vi "InsertBus.vi"(8 "ErrorArray In":errorcluster[](array[cluster]), 11 "BusClass In":refnum<class "Bus.lvclass">) -> (0 "ErrorArray Out":errorcluster[](array[cluster]), 3 "BusClass Out":refnum<class "Bus.lvclass">)   [LabVIEW 2014, in "Bus_class.lvlib" / "Bus.lvclass"]
uses:
  Bus.lvclass
  Bus.lvclass/Bus.ctl
  Framework.lvlib
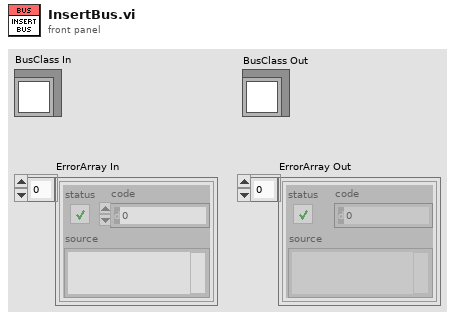
[diagram p1: front panel]
types:
  T1 = typedef "Framework.lvlib/clFrameworkData.ctl" = cluster{"EvtINIFilePaths":path[], "BusClassInstances":refnum<class "Bus.lvclass">[], "PmuImpairINIFilePaths":path[], "FlagImpairINIFilePaths":path[], "NetImpairINIFilePaths":path[], "OutputToFileINIFilePaths":path[], "AppINIFilePaths":path[], "AppModuleID":i32, "OutputToFileID":i32}
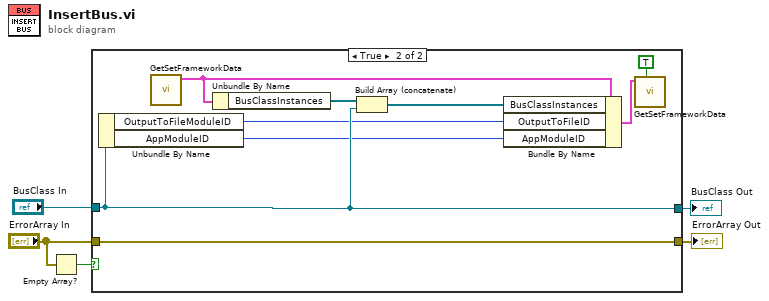
[diagram p0: block diagram]
diagram:
  n1 = Empty Array?(array="ErrorArray In") -> (empty?=w4:bool)
  n2 = case shown="True" w4 {
    tunnel: "ErrorArray In" -> [w6 w13]
    tunnel: "BusClass In" -> [w7 w11]
    tunnel: [w7 w11] -> w2
    tunnel: [w6 w13] -> w1
    frame False {
    }
    frame True {
      n3 = Unbundle By Name(w11) -> ("OutputToFileModuleID"=w9:i32, "AppModuleID"=w8:i32)
      n4 = call "GetSetFrameworkData.vi"() -> ("clFrameworkData Out"=w16:T1)  [unwired: 11 in]
      n5 = Unbundle By Name(w16) -> ("BusClassInstances"=w12:refnum<class "Bus.lvclass">[])
      n6 = Build Array (concatenate)(w12, w11) -> (w10:refnum<class "Bus.lvclass">[])
      n7 = Bundle By Name(cluster=w16, "BusClassInstances"=w10, "OutputToFileID"=w9, "AppModuleID"=w8) -> (w15:T1)
      n8 = call "GetSetFrameworkData.vi"("Set (F)"=TRUE, "clFrameworkData In"=w15) -> ()  [unwired: 9 in, 1 out]
    }
  }
  "BusClass Out" <- w2
  "ErrorArray Out" <- w1
